vi "waveformGraphDraw.vi"(9 "WaveMouse 2":i32, 11 "right wvf graph 2":refnum<vi>) -> (0 "Wavelength 2":dbl caption="Wavelength", 2 "Intensity 2":i32 caption="Intensity")   [LabVIEW 2016]
uses:
  <vilib>/Utility/miscctls.llb/LVPoint32TypeDef.ctl
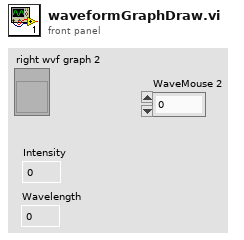
[diagram p1: front panel]
types:
  T1 = cluster{"Width":u16, "Style":enum32{"Solid", "Dash", "Dot", "DashDot", "DashDotDot"}}
  T2 = typedef "LVPoint32TypeDef.ctl" = cluster{"Horizontal":i32, "Vertical":i32}
  T3 = typedef "LVRectTypeDef.ctl" = cluster{"Left":i16, "Top":i16, "Right":i16, "Bottom":i16}
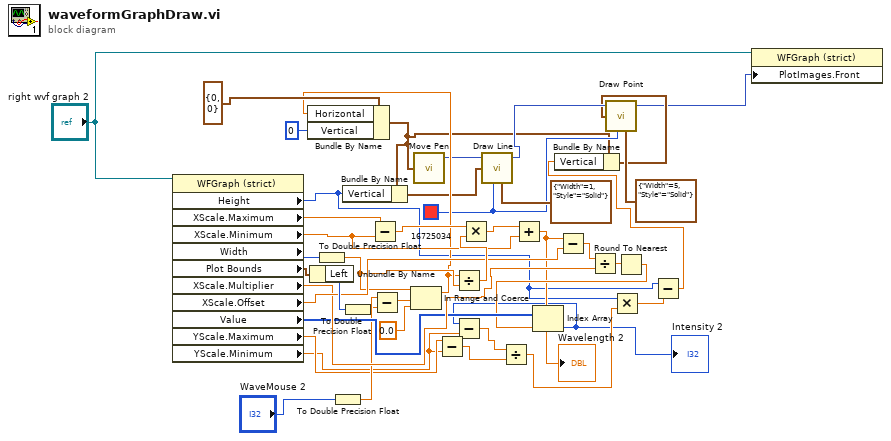
[diagram p0: block diagram]
diagram:
  w11 = u32 16725034 ("color(black)")
  n1 = property class="WFGraph (strict)"(reference="right wvf graph 2") -> ("Height"=w3:u32, "XScale.Maximum"=w38:dbl, "XScale.Minimum"=w34:dbl, "Width"=w39:u32, "Plot Bounds"=w43:T3, "XScale.Multiplier"=w31:dbl, "XScale.Offset"=w33:dbl, "Value"=w29:i32[], "YScale.Maximum"=w16:dbl, "YScale.Minimum"=w4:dbl)  [unwired: 1 in, 2 out]
  n2 = Unbundle By Name(w43) -> ("Left"=w42:i16)
  n3 = To Double Precision Float(number=w39) -> (double precision float=w26:dbl)
  n4 = To Double Precision Float(number="WaveMouse 2") -> (double precision float=w25:dbl)
  n5 = To Double Precision Float(number=w42) -> (double precision float=w24:dbl)
  n6 = Subtract(x=w38, y=w34) -> (x-y=w37:dbl)
  n7 = Subtract(x=w25, y=w24) -> (x-y=w41:dbl)
  n8 = In Range and Coerce(upper limit=w26, x=w41, lower limit=0.0) -> (coerced(x)=w21:dbl)  [unwired: 1 out]
  n9 = Bundle By Name(cluster=T2 {"Horizontal"=0, "Vertical"=0} ("Coords"), "Horizontal"=w21, "Vertical"=0) -> (w10:T2)
  n10 = Bundle By Name(cluster=w10, "Vertical"=w3) -> (w19:T2)
  n11 = call <vilib>:"Move Pen.vi"("new position"=w10) -> ("new picture"=w20:picture)  [unwired: 4 in]
  n12 = Subtract(x=w16, y=w4) -> (x-y=w15:dbl)
  n13 = Divide(x=w21, y=w26) -> (x/y=w36:dbl)
  n14 = Multiply(x=w37, y=w36) -> (x*y=w35:dbl)
  n15 = call <vilib>:"Draw Line.vi"("picture"=w20, "end point"=w19, "color(black)"=w11, "pen"=T1 {"Width"=1, "Style"=enum."Solid"}) -> ("new picture"=w13:picture)  [unwired: 5 in]
  n16 = Add(x=w35, y=w34) -> (x+y=w27:dbl)
  "Wavelength 2" <- w27
  n17 = Subtract(x=w27, y=w33) -> (x-y=w32:dbl)
  n18 = Divide(x=w32, y=w31) -> (x/y=w30:dbl)
  n19 = Round To Nearest(number=w30) -> (nearest integer value=w28:dbl)
  n20 = Index Array(array=w29, index=w28) -> (element=w5:i32)
  "Intensity 2" <- w5
  n21 = Subtract(x=w5, y=w4) -> (x-y=w6:dbl)
  n22 = Divide(x=w6, y=w15) -> (x/y=w14:dbl)
  n23 = Multiply(x=w3, y=w14) -> (x*y=w9:dbl)
  n24 = Subtract(x=w3, y=w9) -> (x-y=w2:dbl)
  n25 = Bundle By Name(cluster=w10, "Vertical"=w2) -> (w8:T2)
  n26 = call <vilib>:"Draw Point.vi"("picture"=w13, "point(x,y)"=w8, "color(black)"=w11, "pen"=T1 {"Width"=5, "Style"=enum."Solid"}) -> ("new picture"=w7:picture)  [unwired: 5 in]
  n27 = property class="WFGraph (strict)"(reference="right wvf graph 2", "PlotImages.Front"=w7) -> ()  [unwired: 1 in, 2 out]
